vi "X+Y.vi"(1 "Y":dbl, 2 "X":dbl) -> (0 "x+y":dbl)   [LabVIEW 2019]
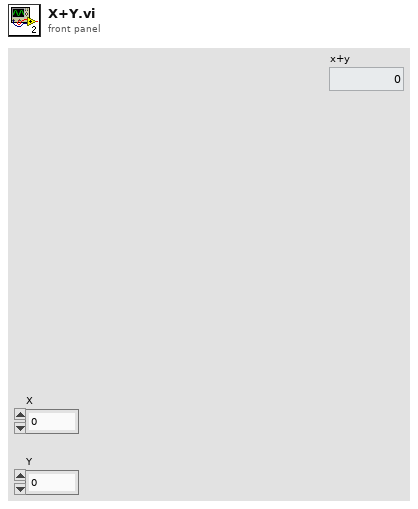
[diagram p1: front panel]
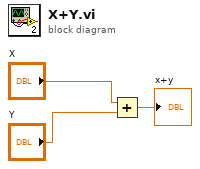
[diagram p0: block diagram]
diagram:
  n1 = Add(x="X", y="Y") -> (x+y=→"x+y":dbl)
